vi "Pass Data Through Tunnels.vi"() -> ()   [LabVIEW 2017]
panel:
  out "Number of Times it Takes to Complete":dbl
  in  "User Picked Value":dbl
  out "Random Number Generated and Rounded":dbl
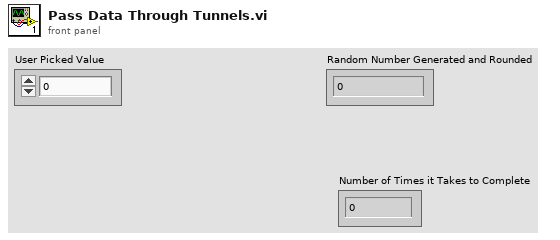
[diagram p1: front panel]
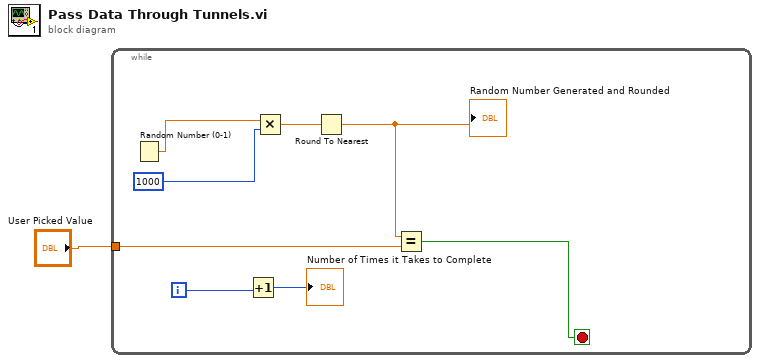
[diagram p0: block diagram]
diagram:
  n1 = while {
    tunnel: "User Picked Value" -> [w9]
    i -> [w6]
    stop <- w8 stop-if-true
    n2 = Random Number (0-1)() -> (number: 0 to 1=w5:dbl)
    n3 = Increment(x=w6) -> (x+1=→"Number of Times it Takes to Complete":i32)
    n4 = Multiply(x=w5, y=1000) -> (x*y=w3:dbl)
    n5 = Round To Nearest(number=w3) -> (nearest integer value=w2:dbl)
    "Random Number Generated and Rounded" <- w2
    n6 = Equal?(x=w2, y=w9) -> (x = y?=w8:bool)
  }
